vi "Stop Nested Actors.vi"(8 "error in (no error)":errorcluster, 11 "Actor with Nesteds in":refnum<class "Actor with Nesteds.lvclass">) -> (0 "error out":errorcluster, 3 "Actor with Nesteds out":refnum<class "Actor with Nesteds.lvclass">)   [LabVIEW 2020, in "Actor with Nesteds.lvlib" / "Actor with Nesteds.lvclass"]
uses:
  Actor with Nesteds.lvclass
  Actor with Nesteds.lvclass/Actor with Nesteds.ctl
  ActorFramework/Actor/Actor.lvclass
  C:/justACS/Actor Framework/Core/ActorFramework/Actor/Actor.lvclass
  C:/justACS/Actor Framework/Core/Testing/Test Harness/Actor with Nesteds/Actor with Nesteds/Actor with Nesteds.lvclass
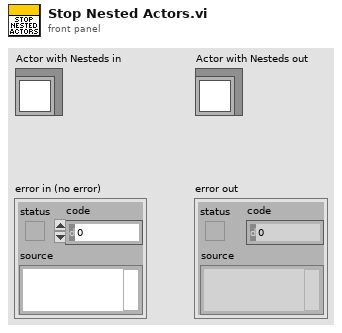
[diagram p1: front panel]
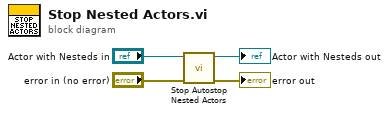
[diagram p0: block diagram]
diagram:
  n1 = call "Stop Autostop Nested Actors.vi"("error in (no error)"="error in (no error)", "Actor in"="Actor with Nesteds in") -> ("error out"=→"error out":errorcluster, "Actor out"=→"Actor with Nesteds out":refnum<class "Actor with Nesteds.lvclass">)  [unwired: 8 in]
